vi "Configure Panel 2.vi"() -> ()   [LabVIEW 2011]
uses:
  UI typedefs/Glue Chuck Control.ctl
  UI typedefs/Glue Slot Control.ctl
  UI typedefs/Stamp Chuck Control.ctl
  UI typedefs/Stamp Slot Control.ctl
  Shared Components/Config Manager Class/Type Definitions/Stamp Type.ctl
  UI typedefs/BBM Chuck Used.ctl
  UI typedefs/Weight Chuck Control.ctl
  UI typedefs/Weight Slot Control.ctl
  Shared Components/Config Manager Class/Type Definitions/Weight Type.ctl
  UI typedefs/BM Chuck Control.ctl
  UI typedefs/BM Slot Control.ctl
  UI typedefs/HDI Chuck Control.ctl
  UI typedefs/HDI Slot Control.ctl
  UI typedefs/Active Paths.ctl
  UI typedefs/Glue Paths.ctl
  UI typedefs/Glue Path.ctl
panel:
  out "Changed":bool
  in  "Glue Pathways":T1=[{"HDI Slot "=0, "Stamp Slot"=0, "Glue Slot"=0, "Weight Slot"=0, "BBM Slot"=0}, {"HDI Slot "=1, "Stamp Slot"=1, "Glue Slot"=1, "Weight Slot"=1, "BBM Slot"=1}, {"HDI Slot "=2, "Stamp Slot"=2, "Glue Slot"=2, "Weight Slot"=2, "BBM Slot"=2}, {"HDI Slot "=3, "Stamp Slot"=3, "Glue Slot"=3, "Weight Slot"=3, "BBM Slot"=3}] {"BBM Slot" items=["Slot 1", "Slot 2", "Slot 3", "Slot 4"]; "Weight Slot" items=["Slot 1", "Slot 2", "Slot 3", "Slot 4"]; "Glue Slot" items=["Slot 1", "Slot 2", "Slot 3", "Slot 4"]; "Stamp Slot" items=["Slot 1", "Slot 2", "Slot 3", "Slot 4"]; "HDI Slot" items=["Slot 1", "Slot 2", "Slot 3", "Slot 4"]}
  out "Active Paths":T3=[TRUE, TRUE, TRUE, TRUE]
  in  "HDI Chuck Control":T4={"Slot 1"={"Populated?"=TRUE, "Identification:"=""}, "Slot 2"={"Populated?"=TRUE, "Identification:"=""}, "Slot 3"={"Populated?"=TRUE, "Identification:"=""}, "Slot 4"={"Populated?"=TRUE, "Identification:"=""}}
  in  "BBM Chuck Control":T6={"Slot 1"={"Populated?"=TRUE}, "Slot 2"={"Populated?"=TRUE}, "Slot 3"={"Populated?"=TRUE}, "Slot 4"={"Populated?"=TRUE}}
  in  "Weight Chuck Control":T8={"Slot 1"={"Populated?"=TRUE, "Weight Type"=enum."Weight 1"}, "Slot 2"={"Populated?"=TRUE, "Weight Type"=enum."Weight 2"}, "Slot 3"={"Populated?"=TRUE, "Weight Type"=enum."Weight 3"}, "Slot 4"={"Populated?"=TRUE, "Weight Type"=enum."Weight 4"}}
  in  "Chuck Module Used for BM:":T11 items=["Chuck 1", "Chuck 2", "Chuck 3", "Chuck 4"]
  in  "Stamp Chuck Control":T12={"Slot 1"={"Populated?"=TRUE, "Stamp Type"=enum."Stamp 1"}, "Slot 2"={"Populated?"=TRUE, "Stamp Type"=enum."Stamp 2"}, "Slot 3"={"Populated?"=TRUE, "Stamp Type"=enum."Stamp 3"}, "Slot 4"={"Populated?"=TRUE, "Stamp Type"=enum."Stamp 4"}}
  in  "Glue Chuck Control":T15={"Slot 1"={"Populated?"=TRUE}, "Slot 2"={"Populated?"=TRUE}, "Slot 3"={"Populated?"=TRUE}, "Slot 4"={"Populated?"=TRUE}}
  in  "Cancel Button":bool
  in  "OK Button":bool
  # "Choose your pathways:"
  # "Procedure:\n1.  Select Chucks that are populated\n2.  Use drop down or text box for identification of element.\n3.  Choose path, as needed."
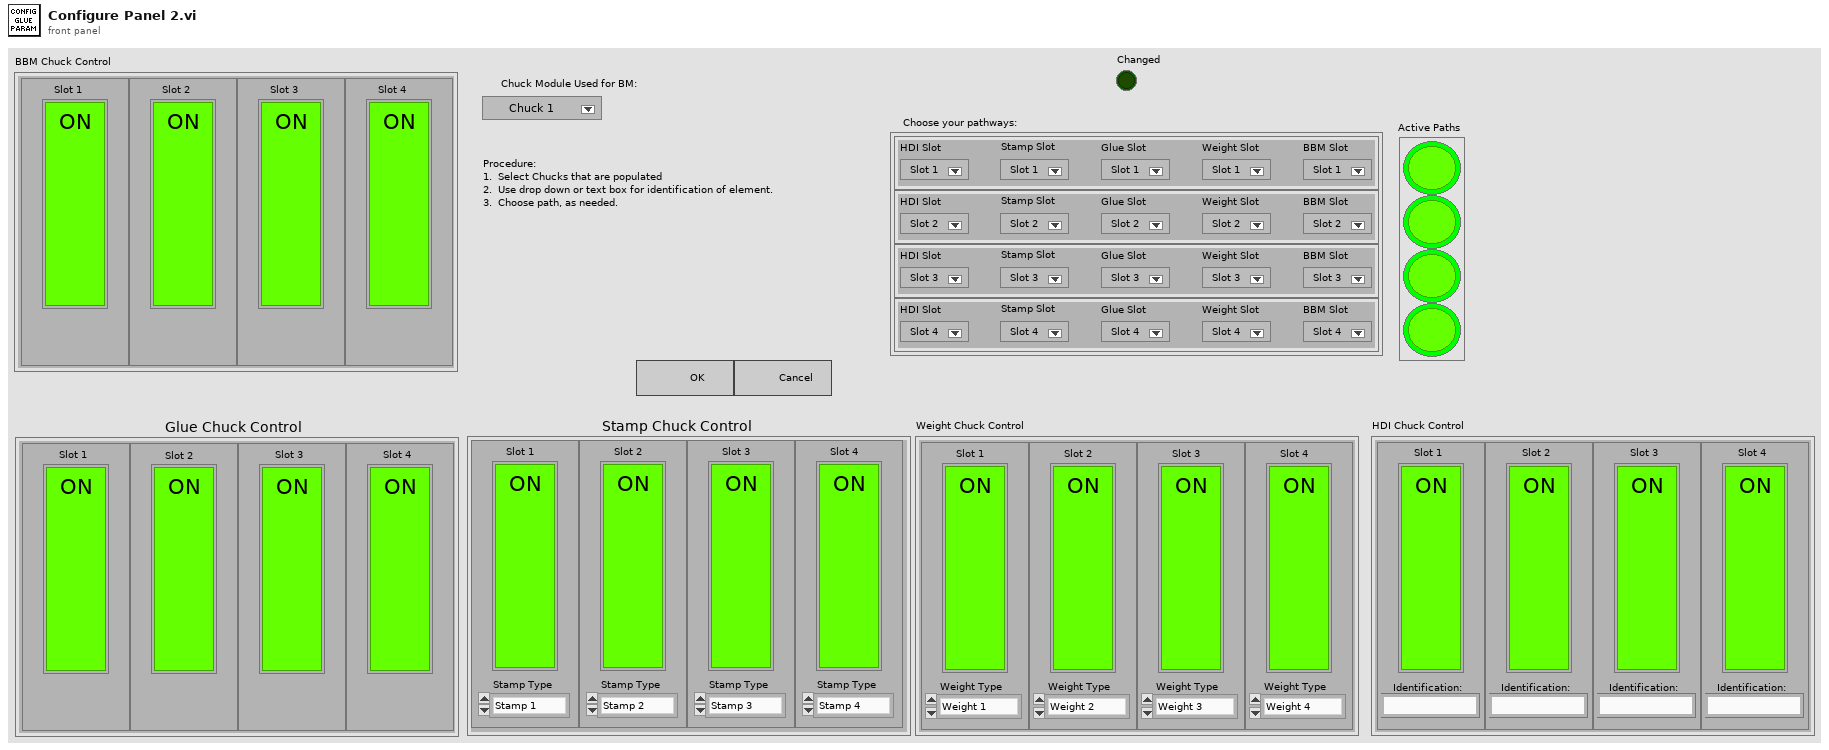
[diagram p1: front panel]
types:
  T1 = typedef "Glue Paths.ctl" = T2[]
  T2 = typedef "Glue Path.ctl" = cluster{"HDI Slot ":i32, "Stamp Slot":u32, "Glue Slot":i32, "Weight Slot":i32, "BBM Slot":i32}
  T3 = typedef "Active Paths.ctl" = bool[]
  T4 = typedef "HDI Chuck Control.ctl" = cluster{"Slot 1":T5, "Slot 2":T5, "Slot 3":T5, "Slot 4":T5}
  T5 = typedef "HDI Slot Control.ctl" = cluster{"Populated?":bool, "Identification:":string}
  T6 = typedef "BM Chuck Control.ctl" = cluster{"Slot 1":T7, "Slot 2":T7, "Slot 3":T7, "Slot 4":T7}
  T7 = typedef "BM Slot Control.ctl" = cluster{"Populated?":bool}
  T8 = typedef "Weight Chuck Control.ctl" = cluster{"Slot 1":T9, "Slot 2":T9, "Slot 3":T9, "Slot 4":T9}
  T9 = typedef "Weight Slot Control.ctl" = cluster{"Populated?":bool, "Weight Type":T10}
  T10 = typedef "Weight Type.ctl" = enum16{"Weight 1", "Weight 2", "Weight 3", "Weight 4", "Weight 5", "Weight 6", "Weight 7", "Weight 8"}
  T11 = typedef "BBM Chuck Used.ctl" = u16
  T12 = typedef "Stamp Chuck Control.ctl" = cluster{"Slot 1":T13, "Slot 2":T13, "Slot 3":T13, "Slot 4":T13}
  T13 = typedef "Stamp Slot Control.ctl" = cluster{"Populated?":bool, "Stamp Type":T14}
  T14 = typedef "Stamp Type.ctl" = enum16{"Stamp 1", "Stamp 2", "Stamp 3", "Stamp 4", "Stamp 5"}
  T15 = typedef "Glue Chuck Control.ctl" = cluster{"Slot 1":T16, "Slot 2":T16, "Slot 3":T16, "Slot 4":T16}
  T16 = typedef "Glue Slot Control.ctl" = cluster{"Populated?":bool}
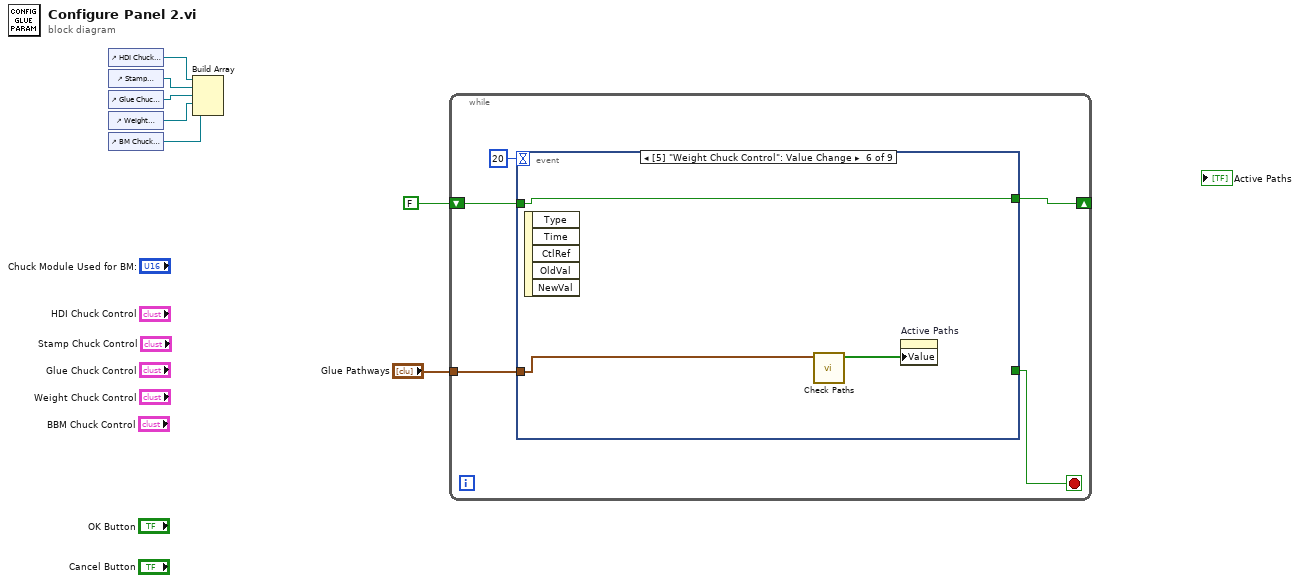
[diagram p0: block diagram]
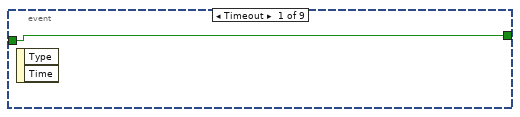
[diagram p2: hidden frame]
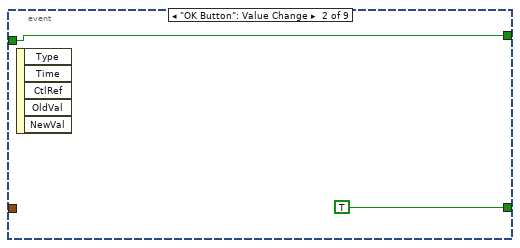
[diagram p3: hidden frame]
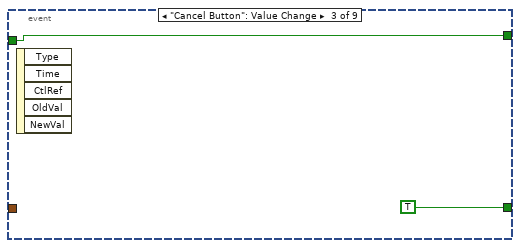
[diagram p4: hidden frame]
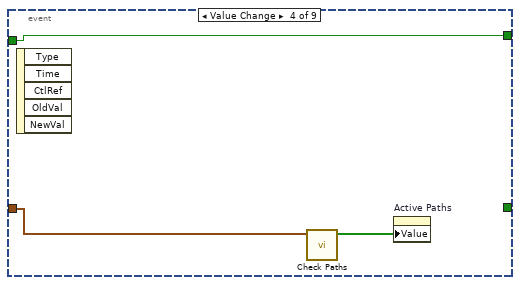
[diagram p5: hidden frame]
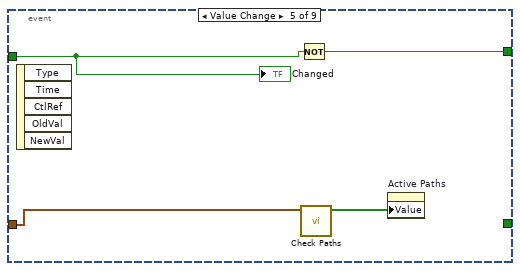
[diagram p6: hidden frame]
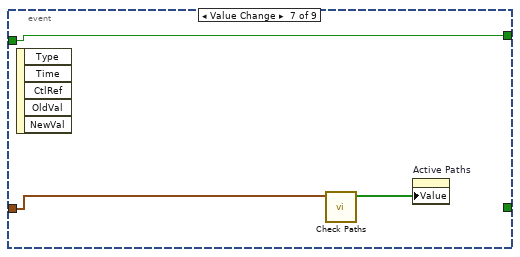
[diagram p7: hidden frame]
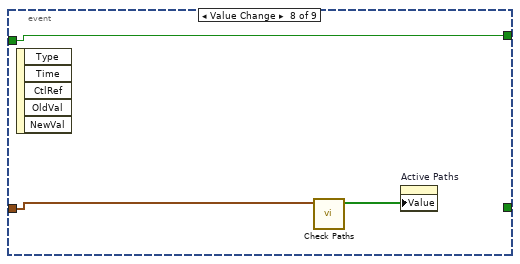
[diagram p8: hidden frame]
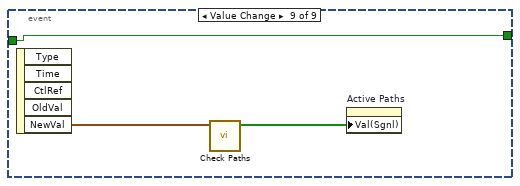
[diagram p9: hidden frame]
diagram:
  n1 = control-ref of="HDI Chuck Control"() -> (w7:refnum<vi>)
  n2 = control-ref of="Stamp Chuck Control"() -> (w6:refnum<vi>)
  n3 = control-ref of="Glue Chuck Control"() -> (w5:refnum<vi>)
  n4 = control-ref of="Weight Chuck Control"() -> (w4:refnum<vi>)
  n5 = control-ref of="BM Chuck Control"() -> (w3:refnum<vi>)
  n6 = Build Array(w7, w6, w5, w4, w3) -> ()  [unwired: 1 out]
  n7 = while {
    tunnel: "Glue Pathways" -> [w11]
    shift-right: [w8] -> _
    shift-left: FALSE ("Changed") -> [w9]
    stop <- w12 stop-if-true
    n8 = event shown="[5] \"Weight Chuck Control\": Value Change" {
      selector: _ -> [_ _ _ _ _ _ _ _ _]
      dyn-events: _ -> [_ _ _ _ _ _ _ _ _]
      timeout: 20 -> [_ _ _ _ _ _ _ _ _]
      tunnel: [_ TRUE TRUE _ _ _ _ _ _] -> w12
      tunnel: w11 -> [_ _ _ w19 w23 w26 w29 w32 _]
      tunnel: w9 -> [w13 w14 w16 w18 w22 w25 w28 w31 w34]
      tunnel: [w13 w14 w16 w18 w21 w25 w28 w31 w34] -> w8
      event Timeout {
        n9 = event-data() -> ()  [unwired: 1 in, 2 out]
      }
      event "OK Button": Value Change {
        n10 = event-data() -> ()  [unwired: 1 in, 5 out]
      }
      event "Cancel Button": Value Change {
        n11 = event-data() -> ()  [unwired: 1 in, 5 out]
      }
      event Value Change {
        n12 = event-data() -> ()  [unwired: 1 in, 5 out]
        n13 = call "Check Paths.vi"("Glue Pathways"=w19) -> ("Active Paths"=w20:T3)  [unwired: 10 in]
        n14 = property on="Active Paths" class="Arr (strict)"("Value"=w20) -> ()  [unwired: 2 in, 2 out]
      }
      event Value Change {
        n15 = event-data() -> ()  [unwired: 1 in, 5 out]
        n16 = Not(x=w22) -> (.not. x?=w21:bool)
        n17 = call "Check Paths.vi"("Glue Pathways"=w23) -> ("Active Paths"=w24:T3)  [unwired: 10 in]
        n18 = property on="Active Paths" class="Arr (strict)"("Value"=w24) -> ()  [unwired: 2 in, 2 out]
        "Changed" <- w22
      }
      event Value Change {
        n19 = event-data() -> ()  [unwired: 1 in, 5 out]
        n20 = call "Check Paths.vi"("Glue Pathways"=w26) -> ("Active Paths"=w27:T3)  [unwired: 10 in]
        n21 = property on="Active Paths" class="Arr (strict)"("Value"=w27) -> ()  [unwired: 2 in, 2 out]
      }
      event Value Change {
        n22 = event-data() -> ()  [unwired: 1 in, 5 out]
        n23 = call "Check Paths.vi"("Glue Pathways"=w29) -> ("Active Paths"=w30:T3)  [unwired: 10 in]
        n24 = property on="Active Paths" class="Arr (strict)"("Value"=w30) -> ()  [unwired: 2 in, 2 out]
      }
      event Value Change {
        n25 = event-data() -> ()  [unwired: 1 in, 5 out]
        n26 = call "Check Paths.vi"("Glue Pathways"=w32) -> ("Active Paths"=w33:T3)  [unwired: 10 in]
        n27 = property on="Active Paths" class="Arr (strict)"("Value"=w33) -> ()  [unwired: 2 in, 2 out]
      }
      event Value Change {
        n28 = event-data() -> ("NewVal"=w36:T1)  [unwired: 1 in, 4 out]
        n29 = call "Check Paths.vi"("Glue Pathways"=w36) -> ("Active Paths"=w35:T3)  [unwired: 10 in]
        n30 = property on="Active Paths" class="Arr (strict)"("Val(Sgnl)"=w35) -> ()  [unwired: 2 in, 2 out]
      }
    }
  }
